vi "VI Name Extract.vi"(11 "VI Refnum":refnum<vi>) -> (3 "Name":string)   [LabVIEW 2023, in "Instruments.lvlib" / "Instruments.lvclass"]
uses:
  Library/Instruments.lvclass
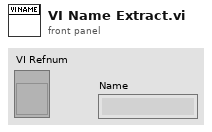
[diagram p1: front panel]
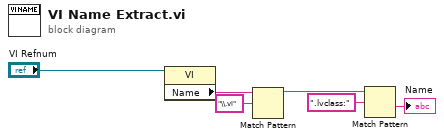
[diagram p0: block diagram]
diagram:
  n1 = property class="VI"(reference="VI Refnum") -> ("Name"=w3:string)  [unwired: 1 in, 2 out]
  n2 = Match Pattern(string=w3, regular expression="\\.vi") -> (before substring=w5:string)  [unwired: 1 in, 3 out]
  n3 = Match Pattern(string=w5, regular expression=".lvclass:") -> (after substring=→"Name":string)  [unwired: 1 in, 3 out]
